vi "DatabseTest_GetRange.vi"() -> ()   [LabVIEW 2015]
uses:
  DatabaseManager/DBManager.lvclass
panel:
  out "Work period":cluster{"Start":timestamp, "End":timestamp}[](array[cluster])
  out "error out":errorcluster
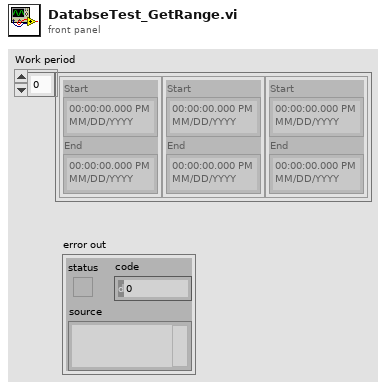
[diagram p1: front panel]
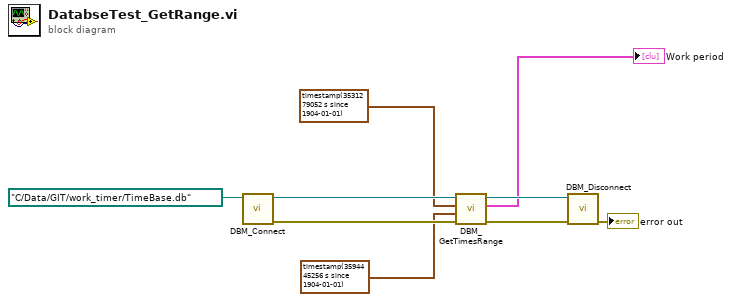
[diagram p0: block diagram]
diagram:
  n1 = call "DBM_Connect.vi"("Path"=path "C:/Data/GIT/work_timer/TimeBase.db") -> ("error out"=w6:errorcluster, "DBManager out"=w7:refnum<class "DBManager.lvclass">)  [unwired: 9 in]
  n2 = call "DBM_GetTimesRange.vi"("error in (no error)"=w6, "End time"=timestamp(3594445256.291 s since 1904-01-01), "Start time"=timestamp(3531279052.395 s since 1904-01-01), "DBManager in"=w7) -> ("error out"=w4:errorcluster, "Work period"=→"Work period":cluster{"Start":timestamp, "End":timestamp}[], "DBManager out"=w5:refnum<class "DBManager.lvclass">)  [unwired: 5 in]
  n3 = call "DBM_Disconnect.vi"("error in (no error)"=w4, "DBManager in"=w5) -> ("error out"=→"error out":errorcluster)  [unwired: 9 in]
